vi "Read MES.vi"(8 "错误输入":errorcluster, 11 "MES路径":path) -> (0 "错误输出":errorcluster, 3 "mes文档":T1)   [LabVIEW 2011]
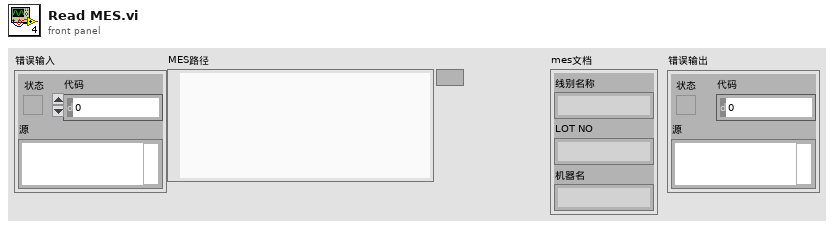
[diagram p1: front panel]
types:
  T1 = cluster{"线别名称":string, "LOT NO":string, "机器名":string}
  T2 = cluster{"IP":string, "PORT":string, "URL":string, "线别名称":string, "LOT NO":string, "机器名":string}
  T3 = cluster{"启用MES":bool, "MES Config":cluster{"SITE":string, "OPERATION":string, "QTY":string, "ACTIVITY":string, "RESOURCE":string, "NC_CODE":string, "IP":string, "PORT":string, "URL":string}}
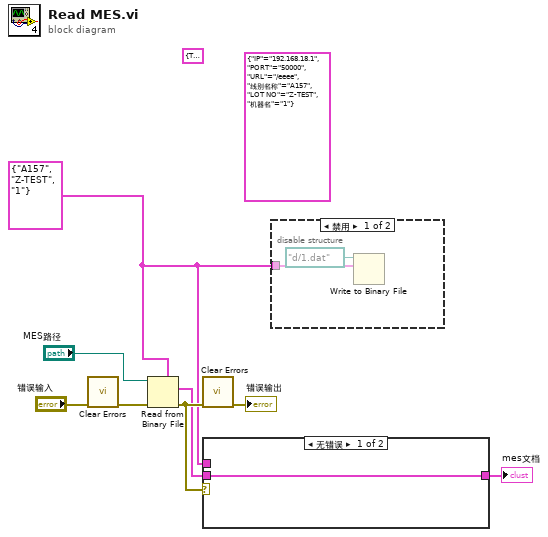
[diagram p0: block diagram]
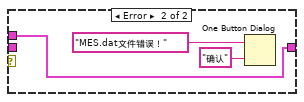
[diagram p3: hidden frame]
diagram:
  w2 = T1 {"线别名称"="A157", "LOT NO"="Z-TEST", "机器名"="1"} ("线别设置")
  (unwired) T2 {"IP"="192.168.18.1", "PORT"="50000", "URL"="/eeee", "线别名称"="A157", "LOT NO"="Z-TEST", "机器名"="1"} ("MES Config")
  (unwired) T3 {"启用MES"=TRUE, "MES Config"={"SITE"="1", "OPERATION"="2", "QTY"="1", "ACTIVITY"="1", "RESOURCE"="1", "NC_CODE"="1", "IP"="192.168.18.1", "PORT"="50000", "URL"="/eeee"}}
  n1 = call <vilib>:"Clear Errors.vi"("error in (no error)"="错误输入") -> ("error out"=w3:errorcluster)  [unwired: 6 in]
  n2 = Read from Binary File(5:w2, 8:w3, 11:"MES路径") -> (0:w5:errorcluster, 2:w4:T1)  [unwired: 3 in, 2 out]
  n3 = call <vilib>:"Clear Errors.vi"("error in (no error)"=w5) -> ("error out"=→"错误输出":errorcluster)  [unwired: 6 in]
  n4 = case shown="无错误" w5 {
    tunnel: [w9 w12] -> w1
    tunnel: w4 -> [w9 _]
    tunnel: w2 -> [_ w12]
    frame No Error {
    }
    frame Error {
      n5 = One Button Dialog(message="MES.dat文件错误！" ("消息"), button name ("OK")="确认" ("按钮名称（“确定”）")) -> ()  [unwired: 1 out]
    }
  }
  "mes文档" <- w1
  n6 = disable-structure shown="禁用" {
    disable-tunnel: w2 -> [w14 _]
    frame Disabled {
      n7 = Write to Binary File(file (use dialog)=path "d:/1.dat" ("文件（使用对话框）"), data=w14) -> ()  [unwired: 4 in, 3 out]
    }
    frame Enabled {
    }
  }
